vi "_Get or Add WorksheetPart.vi"(8 "error in":errorcluster, 11 "SpreadsheetDocument":refnum<k24>) -> (0 "error out":errorcluster, 2 "WorkbookPart":refnum<k24>, 3 "SpreadsheetDocument out":refnum<k24>)   [LabVIEW 2021, in "Open Xml.lvlib"]
uses:
  Open Xml.lvlib
  D:/git/Open-Xml-LabVIEW/dll/DocumentFormat.OpenXml.dll
  dll/DocumentFormat.OpenXml.dll
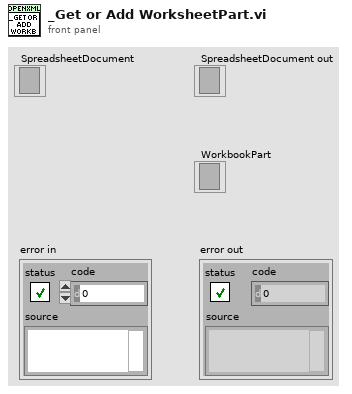
[diagram p1: front panel]
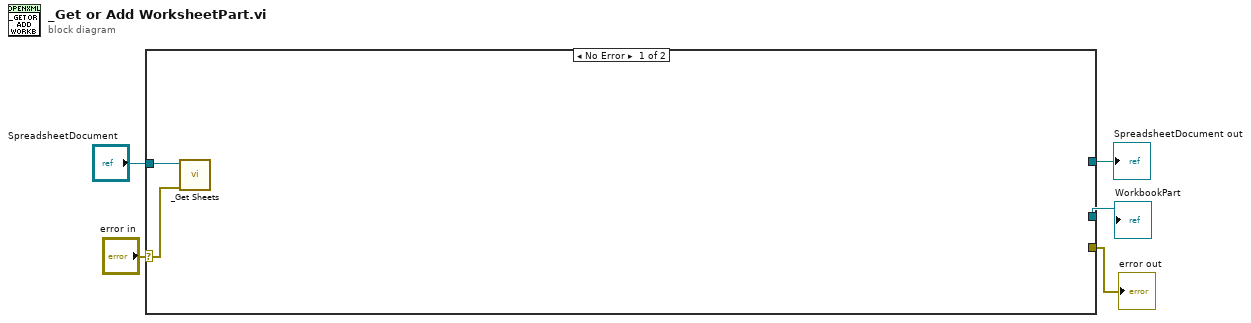
[diagram p0: block diagram]
diagram:
  n1 = case shown="No Error" "error in" {
    selector: "error in" -> [w7 w8]
    tunnel: [_ w8] -> w4
    tunnel: "SpreadsheetDocument" -> [w6 _]
    tunnel: [_ _] -> w2
    tunnel: [_ _] -> w1
    frame No Error {
      n2 = call "_Get Sheets.vi"("error in"=w7, "SpreadsheetDocument in"=w6) -> ()  [unwired: 7 in, 3 out]
    }
    frame Error {
    }
  }
  "error out" <- w4
  "SpreadsheetDocument out" <- w2
  "WorkbookPart" <- w1
